vi "UHR-Fleezers Control (host) - Lorentz v2.vi"() -> ()   [LabVIEW 2014] (continued)
            n459 = local write "Stage Control Serial Error"(w802) -> ()
            n460 = local write "Stage Moving"(TRUE ("Stage Moving")) -> ()
          }
          frame #1 {
            n461 = local write "Stage Moving"(FALSE ("Stage Moving")) -> ()
          }
        }
      }
      event "-x", "+x": Value Change {
        n462 = event-data() -> ()  [unwired: 1 in, 5 out]
        n463 = flat-sequence {
          tunnel: w825 -> [w849]
          tunnel: w826 -> [w833]
          frame #0 {
            n464 = call "Read Stage Position.vi"("error in"=w849, "VISA resource name in"=w833) -> ("Current Position"=w835:cluster{dbl, dbl, dbl}, "error out"=w847:errorcluster, "VISA resource name out"=w848:refnum<visa-resource-name>)  [unwired: 1 out]
            n465 = Divide(x="x nudge increment (um)", y=1000.0) -> (x/y=w846:dbl)
            n466 = Boolean To (0,1)(Boolean="+x") -> (0, 1=w838:i16)
            n467 = Boolean To (0,1)(Boolean="-x") -> (0, 1=w839:i16)
            n468 = Multiply(x=w838, y=w846) -> (x*y=w842:dbl)
            n469 = Multiply(x=w839, y=w846) -> (x*y=w840:dbl)
            n470 = Unbundle(w835) -> (w827:dbl, w829:dbl, w832:dbl)
            n471 = Negate(x=w840) -> (-x=w841:dbl)
            n472 = Add(x=w842, y=w841) -> (x+y=w843:dbl)
            n473 = Add(x=w843, y=w827) -> (x+y=w828:dbl)
            n474 = Bundle(cluster=w835, w828, w829, w832) -> (w834:cluster{dbl, dbl, dbl})
            n475 = call "Set Stage Position.vi"("Position"=w834, "error in"=w847, "VISA resource name in"=w848) -> ("error out"=w830:errorcluster)  [unwired: 2 out]
            n476 = local write "Stage Control Serial Error"(w830) -> ()
            n477 = local write "Stage Moving"(TRUE ("Stage Moving")) -> ()
          }
          frame #1 {
            n478 = local write "Stage Moving"(FALSE ("Stage Moving")) -> ()
          }
        }
      }
      event "Cal/Data Acq. Spot": Value Change {
        # "Disabled by Ronen - we have our own way of controlling the location of calibration."
        n479 = event-data() -> ()  [unwired: 1 in, 5 out]
        n480 = flat-sequence {
          tunnel: w857 -> [w861]
          tunnel: w858 -> [w862]
          tunnel: [w862] -> w854
          tunnel: [w861] -> w853
          tunnel: w854 -> [w865]
          tunnel: w853 -> [w864]
          tunnel: ["Cal @ (MHz)"] -> w851
          tunnel: [w873] -> w855
          tunnel: w851 -> [w873]
          tunnel: w855 -> [w885]
          tunnel: ["W/ Offset 1"] -> w852
          tunnel: w855 -> [w906]
          tunnel: w852 -> [w904]
          frame #0 {
            n481 = property on="Sample Channel\nFlow" class="Bool (strict)"("Val(Sgnl)"="Daq spot flow on") -> ()  [unwired: 2 in, 2 out]
            n482 = Wait (ms)(milliseconds to wait=u32 250) -> ()  [unwired: 1 out]
          }
          frame #1 {
            n483 = disable-structure shown="Disabled" {
              disable-tunnel: w865 -> [w870 _]
              disable-tunnel: w864 -> [w869 _]
              frame Disabled {
                n484 = local read "Saved Stage Positions"() -> (w867:dbl[][])
                n485 = call "move to saved stage position.vi"("error in"=w869, "Stage VISA resource name in"=w870, "Position"="Cal Stage Position", "Saved Stage Positions"=w867) -> ("error out"=w868:errorcluster)  [unwired: 1 out]
                n486 = local write "Stage Control Serial Error"(w868) -> ()
              }
              frame Enabled {
              }
            }
            n487 = property on="Trap Delta (MHz)" class="DigNum (strict)"("Val(Sgnl)"="Cal @ (MHz)") -> ()  [unwired: 2 in, 2 out]
            n488 = local write "Stage Moving"(TRUE ("Stage Moving")) -> ()
          }
          frame #2 {
            n489 = local write "Stage Moving"(FALSE ("Stage Moving")) -> ()
            n490 = property on="Sample Channel\nFlow" class="Bool (strict)"("Val(Sgnl)"="Flow ON during cal?") -> ()  [unwired: 2 in, 2 out]
            n491 = call <vilib>:"Beep.vi"() -> ()  [unwired: 3 in, 9 out]
          }
          frame #3 {
            n492 = Wait (ms)(milliseconds to wait=u32 1000) -> ()  [unwired: 1 out]
          }
          frame #4 {
            n493 = case shown="True" "Active cal after cal?" {
              frame False {
              }
              frame True {
                n494 = local write "Active Cal"(TRUE ("Active Cal")) -> ()
                n495 = Wait (ms)(milliseconds to wait=u32 8000) -> ()  [unwired: 1 out]
              }
            }
          }
          frame #5 {
            n496 = property on="Save Calibration" class="Bool (strict)"("Val(Sgnl)"=TRUE ("Value (Signaling)")) -> ()  [unwired: 2 in, 2 out]
          }
          frame #6 {
            n497 = Wait (ms)(milliseconds to wait=u32 2000) -> ()  [unwired: 1 out]
          }
          frame #7 {
            # "Check to see if \nsaving done"
            n498 = while {
              stop <- w881 stop-if-true
              n499 = local read "Saving..."() -> (w882:bool)
              n500 = Wait (ms)(milliseconds to wait=u32 100) -> ()  [unwired: 1 out]
              n501 = Not(x=w882) -> (.not. x?=w881:bool)
            }
          }
          frame #8 {
            n502 = case shown="True" "W/ Offset 1" {
              tunnel: w885 -> [_ w886]
              frame False {
              }
              frame True {
                n503 = stacked-sequence {
                  tunnel: w886 -> [_ _ _ _ _ _ _ w903]
                  frame #0 {
                    n504 = property on="Trap Delta (MHz)" class="DigNum (strict)"("Val(Sgnl)"="Offset 1 Start (MHz)") -> ()  [unwired: 2 in, 2 out]
                    n505 = Replace Array Subset(array=u32[] [0] ("Index Values"), new element="Offset 1 Set", index=0) -> (w888:u32[])
                    n506 = property on="Saved AOD Raster Scan Parameter Sets" class="Arr (strict)"("Index Values"=w888) -> ()  [unwired: 2 in, 2 out]
                    n507 = property on="manual raster set" class="Ring (strict)"("Value"="Offset 1 Set") -> ()  [unwired: 2 in, 2 out]
                  }
                  frame #1 {
                    n508 = Wait (ms)(milliseconds to wait=u32 200) -> ()  [unwired: 1 out]
                  }
                  frame #2 {
                    n509 = property on="Load parameters" class="Bool (strict)"("Val(Sgnl)"=TRUE ("Value (Signaling)")) -> ()  [unwired: 2 in, 2 out]
                  }
                  frame #3 {
                    n510 = Wait (ms)(milliseconds to wait=u32 200) -> ()  [unwired: 1 out]
                  }
                  frame #4 {
                    n511 = property on="Trap Raster Scan" class="Bool (strict)"("Val(Sgnl)"=TRUE ("Value (Signaling)")) -> ()  [unwired: 2 in, 2 out]
                  }
                  frame #5 {
                    n512 = Wait (ms)(milliseconds to wait=u32 2000) -> ()  [unwired: 1 out]
                  }
                  frame #6 {
                    n513 = while {
                      stop <- w900 stop-if-true
                      n514 = local read "Raster Scanning..."() -> (w902:bool)
                      n515 = local read "Saving..."() -> (w898:bool)
                      n516 = Wait (ms)(milliseconds to wait=u32 100) -> ()  [unwired: 1 out]
                      n517 = Not(x=w898) -> (.not. x?=w897:bool)
                      n518 = Not(x=w902) -> (.not. x?=w899:bool)
                      n519 = And(x=w899, y=w897) -> (x .and. y?=w900:bool)
                    }
                  }
                  frame #7 {
                    n520 = property on="Trap Delta (MHz)" class="DigNum (strict)"("Val(Sgnl)"=w903) -> ()  [unwired: 2 in, 2 out]
                  }
                }
              }
            }
          }
          frame #9 {
            n521 = local read "Save ave N"() -> (w905:dbl)
            n522 = case shown="True" "W/ Offset 2" {
              tunnel: w906 -> [_ w913]
              tunnel: w905 -> [_ w912]
              tunnel: w904 -> [w908 _]
              frame False {
                n523 = case shown="False" w908 {
                  frame False {
                    n524 = Multiply(x="Cal read wait (s)", y=u32 1000 ("milliseconds to wait")) -> (x*y=w910:u32)
                    n525 = Wait (ms)(milliseconds to wait=w910) -> ()  [unwired: 1 out]
                  }
                  frame True {
                  }
                }
              }
              frame True {
                n526 = stacked-sequence {
                  tunnel: w913 -> [_ _ _ _ _ _ _ _ _ w934 _ _]
                  tunnel: w912 -> [_ _ _ _ _ _ _ _ _ w932 _ _]
                  frame #0 {
                    n527 = property on="Save ave N" class="DigNum (strict)"("Val(Sgnl)"=1.0 ("Value (Signaling)")) -> ()  [unwired: 2 in, 2 out]
                  }
                  frame #1 {
                    n528 = Wait (ms)(milliseconds to wait=u32 500) -> ()  [unwired: 1 out]
                  }
                  frame #2 {
                    n529 = property on="Trap Delta (MHz)" class="DigNum (strict)"("Val(Sgnl)"="Offset 2 Start (MHz)") -> ()  [unwired: 2 in, 2 out]
                    n530 = Replace Array Subset(array=u32[] [0] ("Index Values"), new element="Offset 2 Set", index=0) -> (w918:u32[])
                    n531 = property on="Saved AOD Raster Scan Parameter Sets" class="Arr (strict)"("Index Values"=w918) -> ()  [unwired: 2 in, 2 out]
                  }
                  frame #3 {
                    n532 = Wait (ms)(milliseconds to wait=u32 500) -> ()  [unwired: 1 out]
                  }
                  frame #4 {
                    n533 = property on="Load parameters" class="Bool (strict)"("Val(Sgnl)"=TRUE ("Value (Signaling)")) -> ()  [unwired: 2 in, 2 out]
                  }
                  frame #5 {
                    n534 = Wait (ms)(milliseconds to wait=u32 500) -> ()  [unwired: 1 out]
                  }
                  frame #6 {
                    n535 = property on="Trap Raster Scan" class="Bool (strict)"("Val(Sgnl)"=TRUE ("Value (Signaling)")) -> ()  [unwired: 2 in, 2 out]
                  }
                  frame #7 {
                    n536 = Wait (ms)(milliseconds to wait=u32 2000) -> ()  [unwired: 1 out]
                  }
                  frame #8 {
                    n537 = while {
                      stop <- w927 stop-if-true
                      n538 = local read "Raster Scanning..."() -> (w930:bool)
                      n539 = local read "Saving..."() -> (w928:bool)
                      n540 = Wait (ms)(milliseconds to wait=u32 100) -> ()  [unwired: 1 out]
                      n541 = Not(x=w928) -> (.not. x?=w926:bool)
                      n542 = Not(x=w930) -> (.not. x?=w929:bool)
                      n543 = And(x=w929, y=w926) -> (x .and. y?=w927:bool)
                    }
                  }
                  frame #9 {
                    n544 = property on="Trap Delta (MHz)" class="DigNum (strict)"("Val(Sgnl)"=w934) -> ()  [unwired: 2 in, 2 out]
                    n545 = property on="Saved AOD Raster Scan Parameter Sets" class="Arr (strict)"("Index Values"=u32[] [0]) -> ()  [unwired: 2 in, 2 out]
                    n546 = property on="Save ave N" class="DigNum (strict)"("Val(Sgnl)"=w932) -> ()  [unwired: 2 in, 2 out]
                  }
                  frame #10 {
                    n547 = Wait (ms)(milliseconds to wait=u32 500) -> ()  [unwired: 1 out]
                  }
                  frame #11 {
                    n548 = property on="Load parameters" class="Bool (strict)"("Val(Sgnl)"=TRUE ("Value (Signaling)")) -> ()  [unwired: 2 in, 2 out]
                  }
                }
              }
            }
          }
          frame #10 {
            # "Added by Ronen for flow calibration"
            n549 = case shown="True" "Flow based calibration?" {
              frame False {
              }
              frame True {
                n550 = stacked-sequence {
                  frame #0 {
                    n551 = local write "Flow Cal"(TRUE) -> ()
                  }
                  frame #1 {
                  }
                  frame #2 {
                    n552 = Wait (ms)(milliseconds to wait=u32 8000) -> ()  [unwired: 1 out]
                  }
                }
              }
            }
          }
          frame #11 {
            n553 = property on="Read Cal" class="Bool (strict)"("Val(Sgnl)"=TRUE ("Value (Signaling)")) -> ()  [unwired: 2 in, 2 out]
          }
          frame #12 {
            n554 = Wait (ms)(milliseconds to wait=u32 1000) -> ()  [unwired: 1 out]
          }
          frame #13 {
            n555 = property on="Fish for Tether" class="Bool (strict)"("Val(Sgnl)"="Fish after cal?") -> ()  [unwired: 2 in, 2 out]
          }
        }
        n556 = local write "Cal/Data Acq. Spot"(FALSE ("Cal/Data Acq. Spot")) -> ()
      }
      event "Dump Beads": Value Change {
        n557 = event-data() -> ()  [unwired: 1 in, 5 out]
        n558 = flat-sequence {
          tunnel: ["Dump spot flow on?"] -> w943
          tunnel: [w954] -> w944
          tunnel: w943 -> [w954]
          tunnel: w947 -> [w959]
          tunnel: w946 -> [w958]
          tunnel: [w956] -> w945
          tunnel: w944 -> [w956]
          tunnel: w945 -> [w969]
          frame #0 {
            w948 = FALSE ("Value (Signaling)")
            n559 = local read "Saving..."() -> (w950:bool)
            n560 = local write "Dump Beads"(FALSE ("Dump Beads")) -> ()
            n561 = property on="Inject Pump 3" class="Bool (strict)"("Val(Sgnl)"=w948) -> ()  [unwired: 2 in, 2 out]
            n562 = property on="Inject Pump 1" class="Bool (strict)"("Val(Sgnl)"=w948) -> ()  [unwired: 2 in, 2 out]
            n563 = local write "Stop Saving"(w950) -> ()
          }
          frame #1 {
            w951 = FALSE ("Fl. Triggered...")
            n564 = case shown="True" "Dump spot flow on?" {
              frame False {
              }
              frame True {
                n565 = property on="Sample Channel\nFlow" class="Bool (strict)"("Val(Sgnl)"=TRUE ("Stage Moving")) -> ()  [unwired: 2 in, 2 out]
              }
            }
            n566 = local write "Fl. Triggered..."(w951) -> ()
            n567 = local write "Tether"(w951) -> ()
            n568 = property on="Green Laser ON" class="Bool (strict)"("Val(Sgnl)"=w951) -> ()  [unwired: 2 in, 2 out]
            n569 = property on="Trap Pos. FB ON" class="Bool (strict)"("Val(Sgnl)"=w951) -> ()  [unwired: 2 in, 2 out]
            n570 = property on="Trap Trig. Fl." class="Bool (strict)"("Val(Sgnl)"=w951) -> ()  [unwired: 2 in, 2 out]
            n571 = property on="Fl. Triggered..." class="Bool (strict)"("Val(Sgnl)"=w951) -> ()  [unwired: 2 in, 2 out]
            n572 = property on="Dip for Protein" class="Bool (strict)"("Val(Sgnl)"=w951) -> ()  [unwired: 2 in, 2 out]
            n573 = property on="Pause dwell" class="Bool (strict)"("Val(Sgnl)"=w951) -> ()  [unwired: 2 in, 2 out]
          }
          frame #2 {
            n574 = property on="Trap Pos. FB Offset Factor" class="DigNum (strict)"("Val(Sgnl)"=i64 0 ("Value (Signaling)")) -> ()  [unwired: 2 in, 2 out]
          }
          frame #3 {
            n575 = local read "Saved Stage Positions"() -> (w960:dbl[][])
            n576 = local write "Stage Moving"(TRUE ("Stage Moving")) -> ()
            n577 = Array Subset(array=w960, index (row)=3 ("index"), length (row)=1 ("length"), index (col)=1 ("index"), length (col)=3 ("length")) -> (w965:dbl[][])
            n578 = Reshape Array(w965, 3 ("dimension size")) -> (w963:dbl[])
            n579 = Array To Cluster(array=w963) -> (cluster=w962:cluster{"[0]":dbl, "[1]":dbl, "[2]":dbl})
            n580 = call "Set Stage Position.vi"("Position"=w962, "error in"=w958, "VISA resource name in"=w959) -> ()  [unwired: 3 out]
          }
          frame #4 {
            w970 = FALSE ("Value (Signaling)")
            n581 = case shown="True" w969 {
              frame False {
              }
              frame True {
                n582 = property on="Sample Channel\nFlow" class="Bool (strict)"("Val(Sgnl)"=FALSE ("Stage Moving")) -> ()  [unwired: 2 in, 2 out]
              }
            }
            n583 = property on="Trap 1 (ON/OFF)" class="Bool (strict)"("Val(Sgnl)"=w970) -> ()  [unwired: 2 in, 2 out]
            n584 = property on="Trap 2 (ON/OFF)" class="Bool (strict)"("Val(Sgnl)"=w970) -> ()  [unwired: 2 in, 2 out]
            n585 = call <vilib>:"Beep.vi"() -> ()  [unwired: 3 in, 9 out]
          }
          frame #5 {
            n586 = property on="Move Cap. 2 (ADig Top)" class="Bool (strict)"("Val(Sgnl)"=TRUE ("Value (Signaling)")) -> ()  [unwired: 2 in, 2 out]
            n587 = property on="Tab Control" class="TabCtl (strict)"("Val(Sgnl)"=T38."Status" ("Value (Signaling)")) -> ()  [unwired: 2 in, 2 out]
          }
        }
      }
      event "Dip for Protein": Value Change {
        n588 = event-data() -> ()  [unwired: 1 in, 5 out]
        n589 = case shown="True" "Dip for Protein" {
          tunnel: w976 -> [_ w978]
          tunnel: w975 -> [_ w977]
          frame False {
          }
          frame True {
            n590 = while {
              tunnel: w978 -> [w989]
              tunnel: w977 -> [w988]
              i -> [w983]
              stop <- w985 stop-if-true
              n591 = Increment(x=w983) -> (x+1=→"Dip #":i32)
              n592 = flat-sequence {
                tunnel: w988 -> [w1000]
                tunnel: w989 -> [w1001]
                tunnel: [w1001] -> w993
                tunnel: [w1000] -> w992
                tunnel: [w994] -> w979
                tunnel: [w1006] -> w987
                tunnel: [w1007] -> w986
                tunnel: w993 -> [w1008]
                tunnel: w992 -> [w1009]
                tunnel: [w1004] -> w980
                tunnel: w979 -> [w1004]
                tunnel: [w1017] -> w991
                tunnel: w987 -> [w1017]
                tunnel: [w1016] -> w990
                tunnel: w986 -> [w1016]
                tunnel: [w1013] -> w984
                tunnel: [w1012] -> w981
                tunnel: w980 -> [w1012]
                tunnel: w990 -> [w1037]
                tunnel: w991 -> [w1038]
                tunnel: w984 -> [w1039]
                tunnel: w981 -> [w1036]
                tunnel: [w1095] -> w985
                frame #0 {
                  n593 = local read "Trap Pos. FB ON"() -> (w994:bool)
                  n594 = Compound Arithmetic op=AND("Flow ON\nduring dip?", "FB OFF when \nflow ON", w994) -> (w995:bool)
                  n595 = case shown="True" "Move trap \nbefore dip move?" {
                    frame False {
                    }
                    frame True {
                      n596 = property on="Trap Delta (MHz)" class="DigNum (strict)"("Val(Sgnl)"="Dipping Delta (MHz)") -> ()  [unwired: 2 in, 2 out]
                    }
                  }
                  n597 = property on="Green Laser ON" class="Bool (strict)"("Val(Sgnl)"="Green ON\nbefore dip?") -> ()  [unwired: 2 in, 2 out]
                  n598 = property on="Sample Channel\nFlow" class="Bool (strict)"("Val(Sgnl)"="Flow ON\nduring dip?") -> ()  [unwired: 2 in, 2 out]
                  n599 = case shown="True" w995 {
                    frame False {
                    }
                    frame True {
                      n600 = property on="Trap Pos. FB ON" class="Bool (strict)"("Val(Sgnl)"=FALSE ("Value (Signaling)")) -> ()  [unwired: 2 in, 2 out]
                    }
                  }
                }
                frame #1 {
                  n601 = local read "Saved Stage Positions"() -> (w1011:dbl[][])
                  n602 = local write "Cancel dwell"(FALSE ("Cancel dwell")) -> ()
                  n603 = call "move to saved stage position.vi"("error in"=w1009, "Stage VISA resource name in"=w1008, "Position"="Dip Stage \nPosition", "Saved Stage Positions"=w1011) -> ("VISA resource name out"=w1006:refnum<visa-resource-name>, "error out"=w1007:errorcluster)
                }
                frame #2 {
                  n604 = node-c288() -> (w1015:T35)  [unwired: 4 in]
                  n605 = timed-loop {
                    timing: w1015 -> [_]
                    timing-out: [_] -> w1014
                    tunnel: [w1021] -> w1013
                    i -> [w1018]
                    stop <- w1022 stop-if-true
                    n606 = node-c288() -> ()  [unwired: 1 in, 1 out]
                    n607 = Greater Or Equal?(x=w1018, y="Dip Duration (s)") -> (x >= y?=w1030:bool)
                    n608 = local read "Dip for Protein"() -> (w1023:bool)
                    n609 = local read "Dump Beads"() -> (w1020:bool)
                    n610 = local read "Cancel dwell"() -> (w1029:bool)
                    n611 = local read "Pause dwell"() -> (w1026:bool)
                    n612 = Not(x=w1023) -> (.not. x?=w1028:bool)
                    n613 = Compound Arithmetic op=OR(w1029, w1030, w1028) -> (w1027:bool)
                    n614 = Select(t=FALSE, s=w1026, f=w1027) -> (s? t:f=w1024:bool)
                    n615 = Not(x=w1020) -> (.not. x?=w1019:bool)
                    n616 = node-c288() -> ()  [unwired: 1 in, 1 out]
                    n617 = And(x=w1023, y=w1019) -> (x .and. y?=w1021:bool)
                    n618 = Or(x=w1024, y=w1020) -> (x .or. y?=w1022:bool)
                    "Dip Time (s)" <- w1018
                  }
                  n619 = node-c288(w1014) -> ()  [unwired: 1 out]
                }
                frame #3 {
                  n620 = case shown="True" w1039 {
                    tunnel: w1038 -> [_ w1044]
                    tunnel: w1037 -> [_ w1043]
                    tunnel: w1036 -> [_ w1040]
                    frame False {
                    }
                    frame True {
                      n621 = flat-sequence {
                        tunnel: w1043 -> [w1048]
                        tunnel: w1044 -> [w1049]
                        tunnel: [w1049] -> w1042
                        tunnel: [w1048] -> w1041
                        tunnel: w1040 -> [w1045]
                        tunnel: w1042 -> [w1059]
                        tunnel: w1041 -> [w1058]
                        tunnel: w1040 -> [w1067]
                        frame #0 {
                          n622 = local read "Sample Channel\nFlow"() -> (w1047:bool)
                          n623 = case shown="True" w1047 {
                            tunnel: "Flow ON \nduring return\nfrom dip?" -> [w1050 w1053]
                            tunnel: w1045 -> [_ w1052]
                            frame False {
                              n624 = case shown="True" w1050 {
                                frame False {
                                }
                                frame True {
                                n625 = property on="Sample Channel\nFlow" class="Bool (strict)"("Val(Sgnl)"=TRUE ("Value (Signaling)")) -> ()  [unwired: 2 in, 2 out]
                                }
                              }
                            }
                            frame True {
                              n626 = case shown="False" w1053 {
                                tunnel: w1052 -> [w1054 _]
                                frame False {
                                n627 = property on="Trap Pos. FB ON" class="Bool (strict)"("Val(Sgnl)"=w1054) -> ()  [unwired: 2 in, 2 out]
                                n628 = property on="Sample Channel\nFlow" class="Bool (strict)"("Val(Sgnl)"=FALSE ("Value (Signaling)")) -> ()  [unwired: 2 in, 2 out]
                                }
                                frame True {
                                }
                              }
                            }
                          }
                        }
                        frame #1 {
                          # "For turning on green laser before stage reaches lower spot"
                          n629 = case shown="True" "Green ON\nafter start\nreturn?" {
                            frame False {
                            }
                            frame True {
                              n630 = flat-sequence {
                                frame #0 {
                                n631 = Multiply(x="Green delay after \nstart return (s)", y=1000.0) -> (x*y=w1064:dbl)
                                n632 = Wait (ms)(milliseconds to wait=w1064) -> ()  [unwired: 1 out]
                                }
                                frame #1 {
                                n633 = property on="Green Laser ON" class="Bool (strict)"("Val(Sgnl)"=TRUE ("Value (Signaling)")) -> ()  [unwired: 2 in, 2 out]
                                }
                              }
                            }
                          }
                          n634 = local read "Saved Stage Positions"() -> (w1062:dbl[][])
                          n635 = local write "Cancel dwell"(FALSE ("Cancel dwell")) -> ()
                          n636 = call "move to saved stage position.vi"("error in"=w1058, "Stage VISA resource name in"=w1059, "Position"="Return Stage \nPosition", "Saved Stage Positions"=w1062) -> ("error out"=w1060:errorcluster)  [unwired: 1 out]
                          n637 = local write "Stage Control Serial Error"(w1060) -> ()
                        }
                        frame #2 {
                          n638 = property on="Trap Pos. FB ON" class="Bool (strict)"("Val(Sgnl)"=w1067) -> ()  [unwired: 2 in, 2 out]
                          n639 = case shown="True" "Green ON \nafter return?" {
                            frame False {
                            }
                            frame True {
                              n640 = property on="Green Laser ON" class="Bool (strict)"("Val(Sgnl)"=TRUE ("Value (Signaling)")) -> ()  [unwired: 2 in, 2 out]
                            }
                          }
                          n641 = case shown="True" "Move trap after return?" {
                            frame False {
                            }
                            frame True {
                              n642 = property on="Trap Delta (MHz)" class="DigNum (strict)"("Val(Sgnl)"="Dip Trap Delta 2 (MHz)") -> ()  [unwired: 2 in, 2 out]
                            }
                          }
                          n643 = case shown="True" "Save data after return?" {
                            frame False {
                            }
                            frame True {
                              n644 = property on="Start Saving" class="Bool (strict)"("Val(Sgnl)"=TRUE ("Value (Signaling)")) -> ()  [unwired: 2 in, 2 out]
                            }
                          }
                          n645 = property on="Sample Channel\nFlow" class="Bool (strict)"("Val(Sgnl)"="Flow ON\nduring daq?") -> ()  [unwired: 2 in, 2 out]
                        }
                        frame #3 {
                          n646 = node-c288() -> (w1076:T35)  [unwired: 4 in]
                          n647 = timed-loop {
                            timing: w1076 -> [_]
                            timing-out: [_] -> w1075
                            i -> [w1077]
                            stop <- w1079 stop-if-true
                            n648 = node-c288() -> ()  [unwired: 1 in, 1 out]
                            n649 = local read "Dump Beads"() -> (w1078:bool)
                            n650 = Greater Or Equal?(x=w1077, y="Dwell Duration (s)") -> (x >= y?=w1084:bool)
                            n651 = local read "Dip for Protein"() -> (w1081:bool)
                            n652 = Not(x=w1081) -> (.not. x?=w1080:bool)
                            n653 = Compound Arithmetic op=OR(w1084, "Cancel dwell", w1080) -> (w1083:bool)
                            n654 = node-c288() -> ()  [unwired: 1 in, 1 out]
                            n655 = Select(t=FALSE, s="Pause dwell", f=w1083) -> (s? t:f=w1086:bool)
                            n656 = Or(x=w1086, y=w1078) -> (x .or. y?=w1079:bool)
                            "Dwell Time (s)" <- w1077
                          }
                          n657 = node-c288(w1075) -> ()  [unwired: 1 out]
                        }
                      }
                    }
                  }
                }
                frame #4 {
                  n658 = local read "Dip for Protein"() -> (w1096:bool)
                  n659 = local read "Dump Beads"() -> (w1093:bool)
                  n660 = local write "Cancel dwell"(FALSE ("Cancel dwell")) -> ()
                  n661 = Not(x=w1096) -> (.not. x?=w1097:bool)
                  n662 = Not(x="Cont. Repeat Dipping?") -> (.not. x?=w1099:bool)
                  n663 = Compound Arithmetic op=OR(w1097, w1099, w1093) -> (w1095:bool)
                }
              }
            }
          }
        }
      }
      event "Profile": Value Change {
        n664 = event-data() -> ()  [unwired: 1 in, 5 out]
        n665 = flat-sequence {
          tunnel: w1108 -> [w1111]
          tunnel: w1107 -> [w1119]
          tunnel: [w1113] -> w1106
          tunnel: [w1112] -> w1105
          tunnel: [w1110] -> w1103
          tunnel: [w1109] -> w1100
          tunnel: w1106 -> [w1126]
          tunnel: w1105 -> [w1125]
          tunnel: [w1123] -> w1104
          tunnel: w1103 -> [w1124]
          tunnel: [w1122] -> w1102
          tunnel: [w1121] -> w1101
          tunnel: w1100 -> [w1121]
          tunnel: w1104 -> [w1130]
          tunnel: w1102 -> [w1129]
          tunnel: w1101 -> [w1128]
          frame #0 {
            n666 = call "Read Stage Position.vi"("error in"=w1119, "VISA resource name in"=w1111) -> ("Current Position"=w1109:cluster{dbl, dbl, dbl}, "error out"=w1112:errorcluster, "VISA resource name out"=w1110:refnum<visa-resource-name>)  [unwired: 1 out]
            "Current Position" <- w1109
            n667 = local write "Stage Control Serial Error"(w1112) -> ()
            n668 = Unbundle(w1109) -> (w1116:dbl, w1118:dbl, w1114:dbl)
            n669 = Add(x=w1118, y="Y change (mm)") -> (x+y=w1115:dbl)
            n670 = Bundle(w1116, w1115, w1114) -> (w1113:cluster{dbl, dbl, dbl})  [unwired: 1 in]
          }
          frame #1 {
            # "move to new position and start saving"
            n671 = local write "Stage Moving"(TRUE ("Stage Moving")) -> ()
            n672 = local write "Start Saving"(TRUE ("Start Saving")) -> ()
            n673 = call "Set Stage Position.vi"("Position"=w1126, "error in"=w1125, "VISA resource name in"=w1124) -> ("error out"=w1122:errorcluster, "VISA resource name out"=w1123:refnum<visa-resource-name>)  [unwired: 1 out]
          }
          frame #2 {
            # "go back to start"
            n674 = call "Set Stage Position.vi"("Position"=w1128, "error in"=w1129, "VISA resource name in"=w1130) -> ()  [unwired: 3 out]
          }
          frame #3 {
            # "stop saving"
            n675 = local write "Stop Saving"(TRUE ("Stop Saving")) -> ()
            n676 = local write "Stage Moving"(FALSE ("Stage Moving")) -> ()
          }
        }
      }
      event "Move to Position 1", "Move to Position 2", "Move to Position 3", "Move to Position 4", "Move to Position 5", "Lower Ch. Cap.", "Move to Position 6": Value Change {
        n677 = event-data() -> ()  [unwired: 1 in, 5 out]
        n678 = Or(x="Move to Position 5", y="Lower Ch. Cap.") -> (x .or. y?=w1137:bool)
        n679 = Build Array("Move to Position 1", "Move to Position 2", "Move to Position 3", "Move to Position 4", w1137, "Move to Position 6") -> (w1140:bool[])
        n680 = Boolean Array To Number(Boolean array=w1140) -> (number=w1139:u32)
        n681 = Logarithm Base 2(1:w1139) -> (0:w1138:dbl)
        n682 = flat-sequence {
          tunnel: w1138 -> [w1149]
          tunnel: w1135 -> [w1147]
          tunnel: w1134 -> [w1146]
          frame #0 {
            n683 = local read "Saved Stage Positions"() -> (w1157:dbl[][])
            n684 = Array Subset(array=w1157, index (row)=w1149, length (row)=1 ("length"), index (col)=1 ("index"), length (col)=3 ("length")) -> (w1154:dbl[][])
            n685 = Reshape Array(w1154, 3 ("dimension size")) -> (w1152:dbl[])
            n686 = Array To Cluster(array=w1152) -> (cluster=w1151:cluster{"[0]":dbl, "[1]":dbl, "[2]":dbl})
            n687 = call "Set Stage Position.vi"("Position"=w1151, "error in"=w1146, "VISA resource name in"=w1147) -> ("error out"=w1150:errorcluster)  [unwired: 2 out]
            n688 = local write "Stage Moving"(TRUE ("Stage Moving")) -> ()
            n689 = local write "Stage Control Serial Error"(w1150) -> ()
          }
          frame #1 {
            n690 = local write "Stage Moving"(FALSE ("Stage Moving")) -> ()
            n691 = call <vilib>:"Beep.vi"() -> ()  [unwired: 3 in, 9 out]
          }
        }
      }
      event "Got Bead 1": Value Change {
        n692 = event-data() -> ()  [unwired: 1 in, 5 out]
        n693 = flat-sequence {
          tunnel: w1160 -> [w1162]
          tunnel: w1160 -> [w1166]
          frame #0 {
            n694 = for {
              N: w1162 -> [_]
              n695 = property on="Pressure Up" class="Bool (strict)"("Val(Sgnl)"=TRUE) -> ()  [unwired: 2 in, 2 out]
            }
          }
          frame #1 {
          }
          frame #2 {
            n696 = Wait (ms)(milliseconds to wait=u32 1000) -> ()  [unwired: 1 out]
          }
          frame #3 {
          }
          frame #4 {
            n697 = Multiply(x=w1166, y=2) -> (x*y=w1165:i32)
            n698 = for {
              N: w1165 -> [_]
              n699 = property on="Vent pressure" class="Bool (strict)"("Val(Sgnl)"=TRUE) -> ()  [unwired: 2 in, 2 out]
            }
          }
          frame #5 {
            n700 = for {
              N: "Number of Pulses for bead 2" -> [_]
              n701 = property on="Pressure Up" class="Bool (strict)"("Val(Sgnl)"=TRUE) -> ()  [unwired: 2 in, 2 out]
            }
          }
        }
        n702 = local read "Number of pulses For laminar flow"() -> (w1160:i32)
      }
      event "Force FB Data\nScript": Value Change {
        n703 = event-data() -> ()  [unwired: 1 in, 5 out]
        n704 = flat-sequence {
          tunnel: w1176 -> [w1180]
          tunnel: w1177 -> [w1181]
          tunnel: [w1181] -> w1172
          tunnel: [w1180] -> w1171
          tunnel: w1172 -> [w1184]
          tunnel: w1171 -> [w1183]
          tunnel: ["Trap Trig Fl."] -> w1173
          tunnel: [w1209] -> w1174
          tunnel: w1173 -> [w1209]
          tunnel: [w1213] -> w1175
          tunnel: w1174 -> [w1213]
          tunnel: w1175 -> [w1215]
          frame #0 {
            n705 = property on="Trap Delta (MHz)" class="DigNum (strict)"("Val(Sgnl)"="Trap Delta Before Moving") -> ()  [unwired: 2 in, 2 out]
          }
          frame #1 {
            n706 = local read "Saved Stage Positions"() -> (w1186:dbl[][])
            n707 = property on="Trap Pos. FB Offset Factor" class="DigNum (strict)"("Val(Sgnl)"=i64 0 ("Value (Signaling)")) -> ()  [unwired: 2 in, 2 out]
            n708 = local write "FB Trap Pos Offset"(0.0 ("FB Trap Pos Offset")) -> ()
            n709 = local write "Stage Moving"(TRUE ("Stage Moving")) -> ()
            n710 = call "move to saved stage position.vi"("error in"=w1183, "Stage VISA resource name in"=w1184, "Position"="Stage Position To Establish FB", "Saved Stage Positions"=w1186) -> ("error out"=w1182:errorcluster)  [unwired: 1 out]
            n711 = local write "Stage Control Serial Error"(w1182) -> ()
          }
          frame #2 {
            n712 = call <vilib>:"Beep.vi"() -> ()  [unwired: 3 in, 9 out]
            n713 = Multiply(x="Wait (s)", y=u32 1000 ("milliseconds to wait")) -> (x*y=w1193:u32)
            n714 = property on="Trap Delta (MHz)" class="DigNum (strict)"("Val(Sgnl)"="Starting \nTrap Delta (MHz)") -> ()  [unwired: 2 in, 2 out]
            n715 = local write "Stage Moving"(FALSE ("Stage Moving")) -> ()
            n716 = Wait (ms)(milliseconds to wait=w1193) -> ()  [unwired: 1 out]
            n717 = property on="Tab Control 2" class="TabCtl (strict)"("Val(Sgnl)"=T8."Feedback on Trap Position" ("Value (Signaling)")) -> ()  [unwired: 2 in, 2 out]
            n718 = property on="Tab Control" class="TabCtl (strict)"("Val(Sgnl)"=T39."Trap Control (RF)" ("Value (Signaling)")) -> ()  [unwired: 2 in, 2 out]
          }
          frame #3 {
            n719 = property on="Set Reading to\nSetpoint" class="Bool (strict)"("Val(Sgnl)"=TRUE ("Value (Signaling)")) -> ()  [unwired: 2 in, 2 out]
            n720 = Wait (ms)(milliseconds to wait=u32 500) -> ()  [unwired: 1 out]
          }
          frame #4 {
            n721 = property on="Trap Pos. FB ON" class="Bool (strict)"("Val(Sgnl)"=TRUE ("Value (Signaling)")) -> ()  [unwired: 2 in, 2 out]
            n722 = Wait (ms)(milliseconds to wait=u32 250) -> ()  [unwired: 1 out]
          }
          frame #5 {
            n723 = case shown="False" "Trap Trig Fl." {
              frame False {
                n724 = case shown="True" "Green ON after FB ON?" {
                  selector: "Green ON after FB ON?" -> [_ w1208]
                  frame False {
                  }
                  frame True {
                    n725 = property on="Green Laser ON" class="Bool (strict)"("Val(Sgnl)"=w1208) -> ()  [unwired: 2 in, 2 out]
                  }
                }
              }
              frame True {
              }
            }
            n726 = case shown="True" "Remove Action Offset" {
              tunnel: TRUE ("Value (Signaling)") -> [w1205 w1206]
              frame False {
                n727 = property on="Remove Unwinding Offset" class="Bool (strict)"("Val(Sgnl)"=w1205) -> ()  [unwired: 2 in, 2 out]
              }
              frame True {
                n728 = property on="Remove Action Offset" class="Bool (strict)"("Val(Sgnl)"=w1206) -> ()  [unwired: 2 in, 2 out]
              }
            }
            n729 = Wait (ms)(milliseconds to wait=u32 250) -> ()  [unwired: 1 out]
          }
          frame #6 {
            n730 = property on="Start Saving" class="Bool (strict)"("Val(Sgnl)"=TRUE ("Value (Signaling)")) -> ()  [unwired: 2 in, 2 out]
            n731 = Wait (ms)(milliseconds to wait=u32 5000) -> ()  [unwired: 1 out]
          }
          frame #7 {
            w1212 = TRUE ("Value (Signaling)")
            n732 = property on="Rem fb disp offset" class="Bool (strict)"("Val(Sgnl)"=w1212) -> ()  [unwired: 2 in, 2 out]
            n733 = property on="Remove Offset" class="Bool (strict)"("Val(Sgnl)"=w1212) -> ()  [unwired: 2 in, 2 out]
            n734 = Wait (ms)(milliseconds to wait=u32 100) -> ()  [unwired: 1 out]
          }
          frame #8 {
            n735 = case shown="True" w1215 {
              frame False {
              }
              frame True {
                n736 = local write "Trap Trig. Fl."(TRUE ("Value (Signaling)")) -> ()
              }
            }
          }
          frame #9 {
            n737 = case shown="True" "Start dipping after?" {
              frame False {
              }
              frame True {
                n738 = flat-sequence {
                  frame #0 {
                    n739 = Multiply(x="Delay before dipping (s)", y=1000.0) -> (x*y=w1219:dbl)
                    n740 = Wait (ms)(milliseconds to wait=w1219) -> ()  [unwired: 1 out]
                  }
                  frame #1 {
                    n741 = property on="Dip for Protein" class="Bool (strict)"("Val(Sgnl)"=TRUE ("Value (Signaling)")) -> ()  [unwired: 2 in, 2 out]
                    n742 = local write "Scripts"(T1."Dipping" ("Scripts")) -> ()
                  }
                }
              }
            }
          }
        }
      }
      event "Fixed Traps Data\nScript": Value Change {
        n743 = event-data() -> ()  [unwired: 1 in, 5 out]
        n744 = flat-sequence {
          frame #0 {
            n745 = case shown="True" "Green ON" {
              frame False {
              }
              frame True {
                n746 = property on="Green Laser ON" class="Bool (strict)"("Val(Sgnl)"=TRUE) -> ()  [unwired: 2 in, 2 out]
              }
            }
            n747 = local write "Offset (nm)"(0.0 ("Offset (nm)")) -> ()
            n748 = property on="Sample Channel\nFlow" class="Bool (strict)"("Val(Sgnl)"=FALSE ("Value (Signaling)")) -> ()  [unwired: 2 in, 2 out]
            n749 = property on="Trap Delta (MHz)" class="DigNum (strict)"("Val(Sgnl)"="Fixed Traps Trap Delta (MHz)") -> ()  [unwired: 2 in, 2 out]
          }
          frame #1 {
            n750 = Wait (ms)(milliseconds to wait=u32 1000) -> ()  [unwired: 1 out]
          }
          frame #2 {
            n751 = local write "Start Saving"(TRUE ("Start Saving")) -> ()
          }
          frame #3 {
            n752 = local read "Bead Sep. Int. Time (s)"() -> (w1230:dbl)
            n753 = Multiply(x=w1230, y=1000.0) -> (x*y=w1232:dbl)
            n754 = Wait (ms)(milliseconds to wait=w1232) -> ()  [unwired: 1 out]
          }
          frame #4 {
            n755 = property on="Remove Offset" class="Bool (strict)"("Val(Sgnl)"=TRUE ("Value (Signaling)")) -> ()  [unwired: 2 in, 2 out]
          }
          frame #5 {
            n756 = property on="Dip for Protein" class="Bool (strict)"("Val(Sgnl)"="Start dipping after?") -> ()  [unwired: 2 in, 2 out]
          }
        }
      }
      event "Got Bead 2": Value Change {
        # "Got A Dig bead and Got DNA bead events changes by Ronen to Got bead 1 and Got bead 2, and modified to enable operation of the thorlabs motors."
        n757 = event-data() -> ()  [unwired: 1 in, 5 out]
        n758 = flat-sequence {
          tunnel: w1235 -> [w1238]
          frame #0 {
            n759 = case shown="True" "Lumicks Flow During Calibration" {
              tunnel: w1238 -> [_ w1239]
              frame False {
              }
              frame True {
                n760 = for {
                  N: w1239 -> [_]
                  n761 = property on="Pressure Up" class="Bool (strict)"("Val(Sgnl)"=TRUE) -> ()  [unwired: 2 in, 2 out]
                }
              }
            }
          }
          frame #1 {
          }
          frame #2 {
            n762 = Wait (ms)(milliseconds to wait=u32 1000) -> ()  [unwired: 1 out]
          }
          frame #3 {
          }
          frame #4 {
            n763 = case shown="True" "Calibrate after bead 2?" {
              frame False {
              }
              frame True {
                n764 = property on="Cal/Data Acq. Spot" class="Bool (strict)"("Val(Sgnl)"=TRUE) -> ()  [unwired: 2 in, 2 out]
              }
            }
          }
        }
        n765 = local read "Number of pulses For laminar flow"() -> (w1235:i32)
      }
      event "Get New Beads": Value Change {
        # "Flow Control determines how many pressure increases are given when moving."
        n766 = event-data() -> ()  [unwired: 1 in, 6 out]
        n767 = flat-sequence {
          tunnel: w1244 -> [w1246]
          tunnel: w1244 -> [w1250]
          frame #0 {
            n768 = for {
              N: w1246 -> [_]
              n769 = property on="Pressure Up" class="Bool (strict)"("Val(Sgnl)"=TRUE) -> ()  [unwired: 2 in, 2 out]
            }
          }
          frame #1 {
          }
          frame #2 {
            n770 = Wait (ms)(milliseconds to wait=u32 1000) -> ()  [unwired: 1 out]
          }
          frame #3 {
          }
          frame #4 {
            n771 = Multiply(x=2, y=w1250) -> (x*y=w1249:i32)
            n772 = for {
              N: w1249 -> [_]
              n773 = property on="Vent pressure" class="Bool (strict)"("Val(Sgnl)"=TRUE) -> ()  [unwired: 2 in, 2 out]
            }
          }
          frame #5 {
            n774 = for {
              N: "Number of pulses for Bead 1" -> [_]
              n775 = property on="Pressure Up" class="Bool (strict)"("Val(Sgnl)"=TRUE) -> ()  [unwired: 2 in, 2 out]
            }
          }
        }
        n776 = local read "Number of pulses For laminar flow"() -> (w1244:i32)
      }
      event "Take Stepping Data": Value Change {
        n777 = event-data() -> ()  [unwired: 1 in, 5 out]
        n778 = local read "Save ave N"() -> (w1263:dbl)
        n779 = flat-sequence {
          tunnel: w1263 -> [w1265]
          tunnel: [w1265] -> w1258
          tunnel: [w1267] -> w1259
          tunnel: w1258 -> [w1267]
          tunnel: [w1269] -> w1260
          tunnel: w1259 -> [w1269]
          tunnel: [w1272] -> w1261
          tunnel: w1260 -> [w1272]
          tunnel: [w1274] -> w1262
          tunnel: w1261 -> [w1274]
          tunnel: [w1276] -> w1256
          tunnel: w1262 -> [w1276]
          tunnel: w1256 -> [w1279]
          tunnel: [w1279] -> w1255
          tunnel: w1255 -> [w1280]
          tunnel: [w1280] -> w1257
          tunnel: w1257 -> [w1286]
          frame #0 {
            n780 = property on="Save ave N" class="DigNum (strict)"("Val(Sgnl)"="Save ave factor") -> ()  [unwired: 2 in, 2 out]
          }
          frame #1 {
            n781 = Wait (ms)(milliseconds to wait=u32 100) -> ()  [unwired: 1 out]
          }
          frame #2 {
            n782 = local read "Offset 2 Start (MHz)"() -> (w1271:dbl)
            n783 = property on="Saved AOD Raster Scan Parameter Sets" class="Arr (strict)"("Index Values"=u32[] [2]) -> ()  [unwired: 2 in, 2 out]
            n784 = property on="Trap Delta (MHz)" class="DigNum (strict)"("Val(Sgnl)"=w1271) -> ()  [unwired: 2 in, 2 out]
          }
          frame #3 {
            n785 = property on="Load parameters" class="Bool (strict)"("Val(Sgnl)"=TRUE ("Value (Signaling)")) -> ()  [unwired: 2 in, 2 out]
          }
          frame #4 {
            n786 = Wait (ms)(milliseconds to wait=u32 100) -> ()  [unwired: 1 out]
          }
          frame #5 {
            n787 = property on="Trap Raster Scan" class="Bool (strict)"("Val(Sgnl)"=TRUE ("Value (Signaling)")) -> ()  [unwired: 2 in, 2 out]
          }
          frame #6 {
            n788 = Wait (ms)(milliseconds to wait=u32 1000) -> ()  [unwired: 1 out]
          }
          frame #7 {
            n789 = while {
              stop <- w1283 stop-if-true
              n790 = local read "Raster Scanning..."() -> (w1285:bool)
              n791 = local read "Saving..."() -> (w1284:bool)
              n792 = Not(x=w1284) -> (.not. x?=w1281:bool)
              n793 = Not(x=w1285) -> (.not. x?=w1282:bool)
              n794 = And(x=w1282, y=w1281) -> (x .and. y?=w1283:bool)
            }
          }
          frame #8 {
            n795 = property on="Save ave N" class="DigNum (strict)"("Val(Sgnl)"=w1286) -> ()  [unwired: 2 in, 2 out]
          }
        }
      }
      event "Step Size (nm)": Value Change {
        n796 = event-data() -> ()  [unwired: 1 in, 5 out]
        n797 = flat-sequence {
          frame #0 {
            n798 = property on="Saved AOD Raster Scan Parameter Sets" class="Arr (strict)"("Index Values"=u32[] [1]) -> ()  [unwired: 2 in, 2 out]
          }
          frame #1 {
            n799 = Multiply(x="N Steps", y="Step Size (nm)") -> (x*y=w1288:dbl)
            n800 = property on="Scan Speed AOD (nm/s) 2" class="DigNum (strict)"("Value"="Step Size (nm)") -> ()  [unwired: 2 in, 2 out]
            n801 = property on="Step Size AOD (nm) 2" class="DigNum (strict)"("Value"="Step Size (nm)") -> ()  [unwired: 2 in, 2 out]
            n802 = property on="Scan Range AOD (nm) 2" class="DigNum (strict)"("Value"=w1288) -> ()  [unwired: 2 in, 2 out]
          }
        }
      }
      event "Take Detection Laser\nImage": Value Change {
        n803 = event-data() -> ()  [unwired: 1 in, 5 out]
        n804 = flat-sequence {
          tunnel: [w1316] -> w1306
          tunnel: [w1315] -> w1299
          tunnel: [w1314] -> w1291
          tunnel: [w1319] -> w1307
          tunnel: w1306 -> [w1319]
          tunnel: [w1318] -> w1300
          tunnel: w1299 -> [w1318]
          tunnel: [w1317] -> w1292
          tunnel: w1291 -> [w1317]
          tunnel: [w1323] -> w1308
          tunnel: w1307 -> [w1323]
          tunnel: [w1322] -> w1301
          tunnel: w1300 -> [w1322]
          tunnel: [w1321] -> w1293
          tunnel: w1292 -> [w1321]
          tunnel: [w1329] -> w1309
          tunnel: w1308 -> [w1329]
          tunnel: [w1328] -> w1302
          tunnel: w1301 -> [w1328]
          tunnel: [w1327] -> w1294
          tunnel: w1293 -> [w1327]
          tunnel: [w1333] -> w1310
          tunnel: w1309 -> [w1333]
          tunnel: [w1332] -> w1303
          tunnel: w1302 -> [w1332]
          tunnel: [w1331] -> w1295
          tunnel: w1294 -> [w1331]
          tunnel: [w1337] -> w1311
          tunnel: w1310 -> [w1337]
          tunnel: [w1336] -> w1304
          tunnel: w1303 -> [w1336]
          tunnel: [w1335] -> w1296
          tunnel: w1295 -> [w1335]
          tunnel: [w1341] -> w1312
          tunnel: w1311 -> [w1341]
          tunnel: [w1340] -> w1305
          tunnel: w1304 -> [w1340]
          tunnel: [w1339] -> w1297
          tunnel: w1296 -> [w1339]
          tunnel: w1312 -> [w1347]
          tunnel: w1305 -> [w1346]
          tunnel: [w1344] -> w1298
          tunnel: w1297 -> [w1344]
          tunnel: w1298 -> [w1348]
          frame #0 {
            n805 = local read "Laser interlacing mode"() -> (w1315:enum32{"Laser ON", "Laser OFF", "Interlace"})
            n806 = local read "Green FB On/Off"() -> (w1314:bool)
            n807 = local read "Green Laser ON"() -> (w1316:bool)
          }
          frame #1 {
            n808 = property on="Green FB On/Off" class="Bool (strict)"("Val(Sgnl)"=FALSE ("Value (Signaling)")) -> ()  [unwired: 2 in, 2 out]
          }
          frame #2 {
            n809 = property on="Green Laser ON" class="Bool (strict)"("Val(Sgnl)"=TRUE ("Value (Signaling)")) -> ()  [unwired: 2 in, 2 out]
            n810 = property on="Flip Green Filter" class="Bool (strict)"("Val(Sgnl)"=TRUE ("Value (Signaling)")) -> ()  [unwired: 2 in, 2 out]
            n811 = property on="Laser interlacing mode" class="RadioBtnsControl (strict)"("Val(Sgnl)"=enum32{"Laser ON", "Laser OFF", "Interlace"}."Laser ON" ("Value (Signaling)")) -> ()  [unwired: 2 in, 2 out]
          }
          frame #3 {
            n812 = Wait (ms)(milliseconds to wait=u32 500) -> ()  [unwired: 1 out]
          }
          frame #4 {
            n813 = property on="Confocal Image" class="Bool (strict)"("Val(Sgnl)"=TRUE ("Value (Signaling)")) -> ()  [unwired: 2 in, 2 out]
          }
          frame #5 {
            n814 = Wait (ms)(milliseconds to wait=u32 2000) -> ()  [unwired: 1 out]
          }
          frame #6 {
            n815 = while {
              stop <- w1342 stop-if-true
              n816 = local read "Saving..."() -> (w1343:bool)
              n817 = Not(x=w1343) -> (.not. x?=w1342:bool)
            }
          }
          frame #7 {
            n818 = property on="Flip Green Filter" class="Bool (strict)"("Val(Sgnl)"=TRUE ("Value (Signaling)")) -> ()  [unwired: 2 in, 2 out]
            n819 = property on="Green Laser ON" class="Bool (strict)"("Val(Sgnl)"=w1347) -> ()  [unwired: 2 in, 2 out]
            n820 = property on="Laser interlacing mode" class="RadioBtnsControl (strict)"("Val(Sgnl)"=w1346) -> ()  [unwired: 2 in, 2 out]
          }
          frame #8 {
            n821 = property on="Green FB On/Off" class="Bool (strict)"("Val(Sgnl)"=w1348) -> ()  [unwired: 2 in, 2 out]
          }
        }
      }
      event "Move in a Circle": Value Change {
        w1350 = dbl[] []
        # "converting distance (d) to angle (a)\na=arcsin(d/2r)"
        # "radius"
        # "radius"
        # "T1 Y"
        # "T1 X"
        n822 = event-data() -> ()  [unwired: 1 in, 5 out]
        n823 = local read "BD 1 Frequency 1 (MHz)"() -> (w1358:dbl)
        n824 = local read "BD 2 Frequency 1 (MHz)"() -> (w1357:dbl)
        n825 = local read "BD 1 Frequency 2 (MHz)"() -> (w1356:dbl)
        n826 = local read "BD 2 Frequency 2 (MHz)"() -> (w1355:dbl)
        n827 = Subtract(x=w1357, y="Center Y Frequency (MHz)") -> (x-y=w1362:dbl)
        n828 = Absolute Value(x=w1362) -> (abs(x)=w1353:dbl)
        n829 = flat-sequence {
          tunnel: w1353 -> [w1365]
          tunnel: [w1365] -> w1352
          frame #0 {
            n830 = local write "Radius (MHz)"(w1365) -> ()
          }
        }
        n831 = node-c288("Time step (ms)") -> (w1364:T35)  [unwired: 3 in]
        n832 = timed-loop {
          timing: w1364 -> [_]
          timing-out: [_] -> w1363
          tunnel: w1358 -> [w1456]
          tunnel: w1357 -> [_]
          tunnel: w1356 -> [w1460]
          tunnel: w1355 -> [_]
          tunnel: "Center Y Frequency (MHz)" -> [w1449]
          shift-right: [w1410] -> _
          shift-left: w1350 -> [w1417]
          shift-right: [w1408] -> _
          shift-left: w1350 -> [w1416]
          shift-right: [w1401] -> _
          shift-left: w1350 -> [w1414]
          shift-right: [w1399] -> _
          shift-left: w1350 -> [w1413]
          tunnel: "Move in a Circle" -> [_]
          tunnel: ["Back to start on finish?"] -> w1354
          tunnel: w1352 -> [_]
          tunnel: w1351 -> [w1431]
          tunnel: w1350 -> [w1412]
